vi "Conditional Auto-Indexing Tunnel__ogtk.vi"   [LabVIEW 2014]
doc: "This polymorphic VI filters <B>Array In</B> by keeping only those elements where corresponding elements in <B>Elements to keep</B> are TRUE."
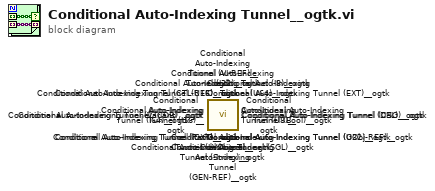
[diagram p0: block diagram]
diagram:
  n1 = call <userlib>:"Conditional Auto-Indexing Tunnel (LVObject)__ogtk.vi"() -> ()  [unwired: 7 in, 1 out]
  n2 = call <userlib>:"Conditional Auto-Indexing Tunnel (U64)__ogtk.vi"() -> ()  [unwired: 7 in, 1 out]
  n3 = call <userlib>:"Conditional Auto-Indexing Tunnel (I64)__ogtk.vi"() -> ()  [unwired: 7 in, 1 out]
  n4 = call <userlib>:"Conditional Auto-Indexing Tunnel (Bool)__ogtk.vi"() -> ()  [unwired: 7 in, 1 out]
  n5 = call <userlib>:"Conditional Auto-Indexing Tunnel (CTL-REF)__ogtk.vi"() -> ()  [unwired: 7 in, 1 out]
  n6 = call <userlib>:"Conditional Auto-Indexing Tunnel (VI-REF)__ogtk.vi"() -> ()  [unwired: 7 in, 1 out]
  n7 = call <userlib>:"Conditional Auto-Indexing Tunnel (GObj-REF)__ogtk.vi"() -> ()  [unwired: 7 in, 1 out]
  n8 = call <userlib>:"Conditional Auto-Indexing Tunnel (GEN-REF)__ogtk.vi"() -> ()  [unwired: 7 in, 1 out]
  n9 = call <userlib>:"Conditional Auto-Indexing Tunnel (CXT)__ogtk.vi"() -> ()  [unwired: 7 in, 1 out]
  n10 = call <userlib>:"Conditional Auto-Indexing Tunnel (CDB)__ogtk.vi"() -> ()  [unwired: 7 in, 1 out]
  n11 = call <userlib>:"Conditional Auto-Indexing Tunnel (CSG)__ogtk.vi"() -> ()  [unwired: 7 in, 1 out]
  n12 = call <userlib>:"Conditional Auto-Indexing Tunnel (EXT)__ogtk.vi"() -> ()  [unwired: 7 in, 1 out]
  n13 = call <userlib>:"Conditional Auto-Indexing Tunnel (SGL)__ogtk.vi"() -> ()  [unwired: 7 in, 1 out]
  n14 = call <userlib>:"Conditional Auto-Indexing Tunnel (I8)__ogtk.vi"() -> ()  [unwired: 7 in, 1 out]
  n15 = call <userlib>:"Conditional Auto-Indexing Tunnel (I16)__ogtk.vi"() -> ()  [unwired: 7 in, 1 out]
  n16 = call <userlib>:"Conditional Auto-Indexing Tunnel (U8)__ogtk.vi"() -> ()  [unwired: 7 in, 1 out]
  n17 = call <userlib>:"Conditional Auto-Indexing Tunnel (U16)__ogtk.vi"() -> ()  [unwired: 7 in, 1 out]
  n18 = call <userlib>:"Conditional Auto-Indexing Tunnel (U32)__ogtk.vi"() -> ()  [unwired: 7 in, 1 out]
  n19 = call <userlib>:"Conditional Auto-Indexing Tunnel (I32)__ogtk.vi"() -> ()  [unwired: 7 in, 1 out]
  n20 = call <userlib>:"Conditional Auto-Indexing Tunnel (Path)__ogtk.vi"() -> ()  [unwired: 7 in, 1 out]
  n21 = call <userlib>:"Conditional Auto-Indexing Tunnel (DBL)__ogtk.vi"() -> ()  [unwired: 7 in, 1 out]
  n22 = call <userlib>:"Conditional Auto-Indexing Tunnel (String)__ogtk.vi"() -> ()  [unwired: 7 in, 1 out]
  n23 = call <userlib>:"Conditional Auto-Indexing Tunnel (Variant)__ogtk.vi"() -> ()  [unwired: 7 in, 1 out]
